vi "Teleop.vi"(10 "Match Info":T1={"Autonomous Elapsed Seconds"=0.0, "TeleOp Elapsed Seconds"=0.0, "Disabled Elapsed Seconds"=0.0, "Visited Autonomous"=FALSE, "Visited TeleOp"=FALSE, "Visited Disabled"=FALSE, "Autonomous Settings"={"Autonomous Style"=enum."Independent", "VI Refnum"=refnum}}, 11 "Call Context":T2) -> ()   [LabVIEW 2012]
doc: "This VI is called for each TeleOp packet received from the DS where the robot is not disabled. It is often used to read from the joysticks and update I/O or to update setpoints for timed control loops. It should complete and return within 20 milliseconds or it may miss DS packets."
uses:
  <vilib>/Rock Robotics/WPI/DriverStation/WPI_DriverStationDerivedRobotMode.ctl
  <vilib>/Rock Robotics/WPI/DriverStation/WPI_DriverStationMatch Info.ctl
  Robot Global Data.vi
  <vilib>/Rock Robotics/WPI/RobotDrive/WPI_RobotDriveGetSetRefNum.vi
panel:
  in  "Feeder Angle On Cannon In Minimum Position":dbl
  in  "Feeder Sit On Cannon?":bool=TRUE
  out "Cannon Angle (Relative to the Horizon)":dbl
  in  "reset":bool
  in  "Telescopic Toghether?":bool
  in  "Cannons Toghether?":bool
  in  "Cananot Toghether?":bool
  in  "2  Cananot (Climb)":dbl(slide) scale=-1.0..1.0
  in  "2  Telescopic(Climb)":dbl(slide) scale=-1.0..1.0
  in  "2 Cannons":dbl(slide) scale=-1.0..1.0
  in  "Flipper Servos":i32(knob) scale=0.0..170.0
  in  "Feeder Servos":i32(knob) scale=0.0..160.0
  in  "Climb Telescopic Right":dbl(slide) scale=-1.0..1.0
  in  "Climb Telescopic Left":dbl(slide) scale=-1.0..1.0
  in  "Transfer":dbl(slide) scale=-1.0..1.0
  in  "Canenet Left":dbl(slide) scale=-1.0..1.0
  in  "Canenet Right":dbl(slide) scale=-1.0..1.0
  in  "Conveyer Belt":dbl(slide) scale=-1.0..1.0
  in  "zAvit":dbl(slide) scale=-1.0..1.0
  in  "First Cannon":dbl(slide) scale=-1.0..1.0
  in  "Second Cannon":dbl(slide) scale=-1.0..1.0
  in  "Y axis value":dbl(slide) scale=-1.0..1.0
  in  "X axis value":dbl(slide) scale=-1.0..1.0
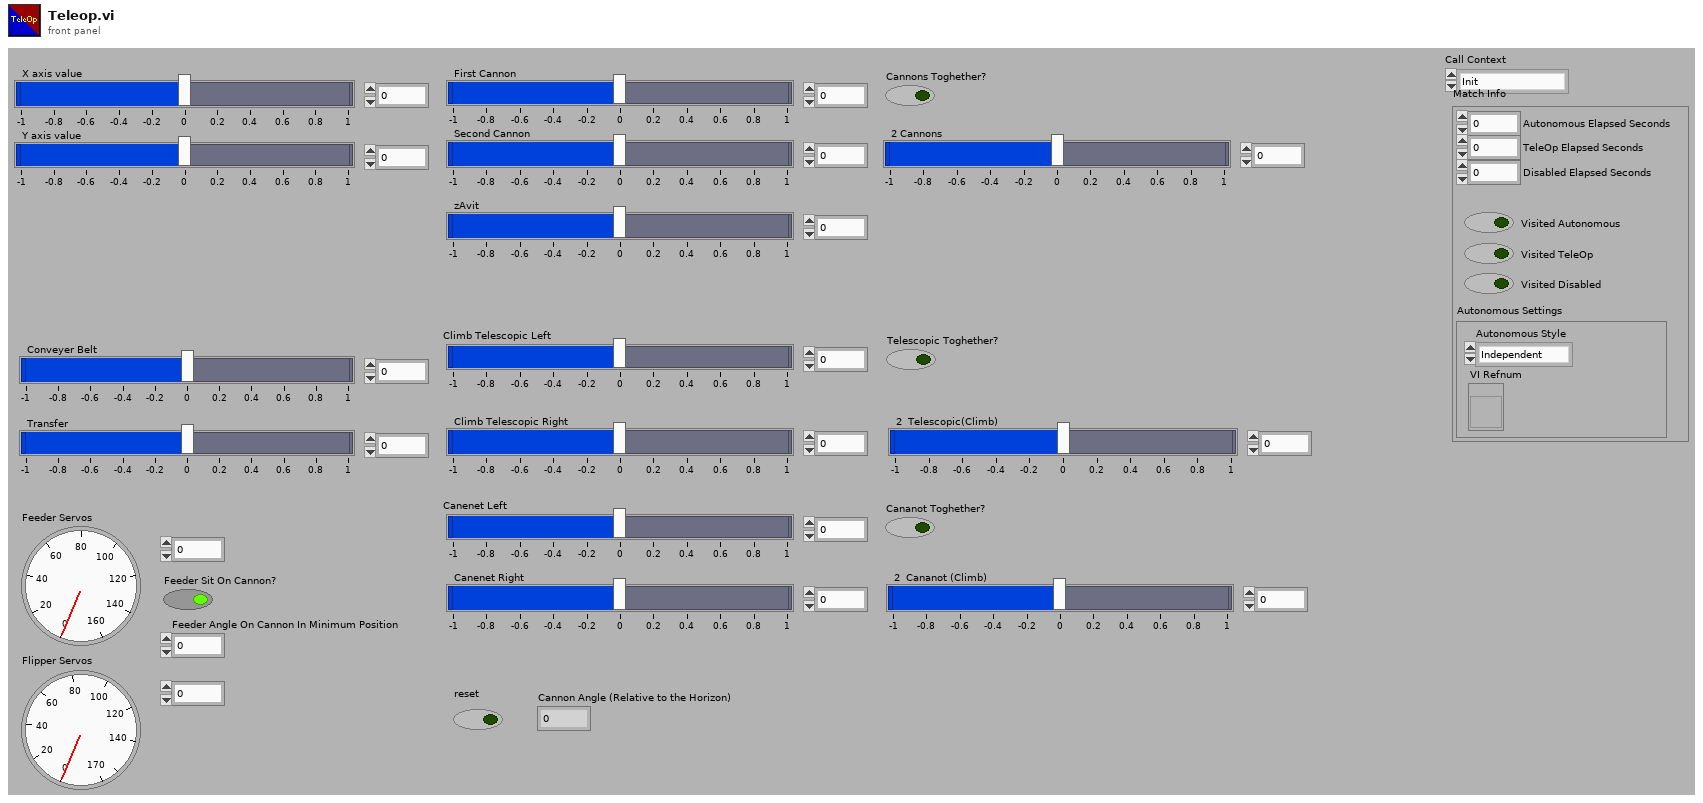
[diagram p1: front panel]
types:
  T1 = typedef "WPI_DriverStationMatch Info.ctl" = cluster{"Autonomous Elapsed Seconds":dbl, "TeleOp Elapsed Seconds":dbl, "Disabled Elapsed Seconds":dbl, "Visited Autonomous":bool, "Visited TeleOp":bool, "Visited Disabled":bool, "Autonomous Settings":cluster{"Autonomous Style":enum16{"Iterative", "Independent"}, "VI Refnum":refnum<vi>}}
  T2 = typedef "WPI_DriverStationDerivedRobotMode.ctl" = enum16{"Init", "Execute", "Stop"}
  T3 = typedef "WPI_AnalogChannelDevRef.ctl" = cluster{"DevStatus":errorcluster, "Analog Module":T4, "Analog Channel":T5}
  T4 = typedef "FPGA_TypedefAnalogModule.ctl" = enum16{"Analog Module 1", "Analog Module 2"}
  T5 = typedef "FPGA_AIChannel.ctl" = enum8{"AI 1", "AI 2", "AI 3", "AI 4", "AI 5", "AI 6", "AI 7", "AI 8", "Invalid"}
  T6 = typedef "WPI_DigitalInputDevRef.ctl" = cluster{"DevStatus":errorcluster, "DIO Channel":T7, "Digital Module":T8}
  T7 = typedef "FPGA_DIOChannel.ctl" = enum8{"DIO 1", "DIO 2", "DIO 3", "DIO 4", "DIO 5", "DIO 6", "DIO 7", "DIO 8", "DIO 9", "DIO 10", "DIO 11", "DIO 12", "DIO 13", "DIO 14", "Invalid"}
  T8 = typedef "FPGA_TypedefDigitalModule.ctl" = enum16{"Digital Module 1", "Digital Module 2"}
  T9 = typedef "WPI_MotorControlDeviceRef.ctl" = cluster{"DeviceStatus":errorcluster, "Type":enum16{"PWM", "CAN"}, "PWM":cluster{"Digital Module":T8, "PWM Channel":T10, "DeadBand":T11}, "CAN":cluster{"Device Number":u8, "Control Mode":T12, "Semaphore":T13, "Max Vout":dbl}, "Invert":bool, "TransformRef":T14, "InvTransformRef":T14}
  T10 = typedef "FPGA_DIOPWMChannel.ctl" = enum8{"PWM 1", "PWM 2", "PWM 3", "PWM 4", "PWM 5", "PWM 6", "PWM 7", "PWM 8", "PWM 9", "PWM 10", "Invalid"}
  T11 = typedef "WPI_PWMDeadband.ctl" = cluster{"Name":string, "maxPositivePwm":i32, "minPositivePwm":i32, "centerPwm":i32, "maxNegativePwm":i32, "minNegativePwm":i32, "angularRange":u16}
  T12 = typedef "WPI_CANJaguar_ControlMode.ctl" = enum8{"Percent VBus", "Current", "Speed", "Position", "Voltage"}
  T13 = typedef "Semaphore RefNum" = refnum<k1>
  T14 = typedef "WPI_PWMTransform_ConPane.ctl" = refnum<vi>
  T15 = typedef "WPI_ServoDeviceRef.ctl" = cluster{"DeviceStatus":errorcluster, "Digital Module":T8, "PWM Channel":T10, "DeadBand":T11}
  T16 = typedef "WPI_RobotDriveDevRef.ctl" = cluster{"DevStatus":errorcluster, "Motors[]":T9[], "Square Inputs":bool, "Max Output":dbl, "Isochronous":bool}
  T17 = typedef "WPI_RelayDevRef.ctl" = cluster{"DevStatus":errorcluster, "Relay Channel":T18, "Digital Module":T8, "Relay Direction":T19}
  T18 = typedef "FPGA_DIORelayChannel.ctl" = enum8{"Relay 1", "Relay 2", "Relay 3", "Relay 4", "Relay 5", "Relay 6", "Relay 7", "Relay 8", "Invalid"}
  T19 = typedef "WPI_RelayDirection.ctl" = enum16{"Both directions", "Forward only", "Reverse only"}
  T20 = typedef "WPI_RelayValue.ctl" = enum16{"Off", "On", "Forward", "Reverse"}
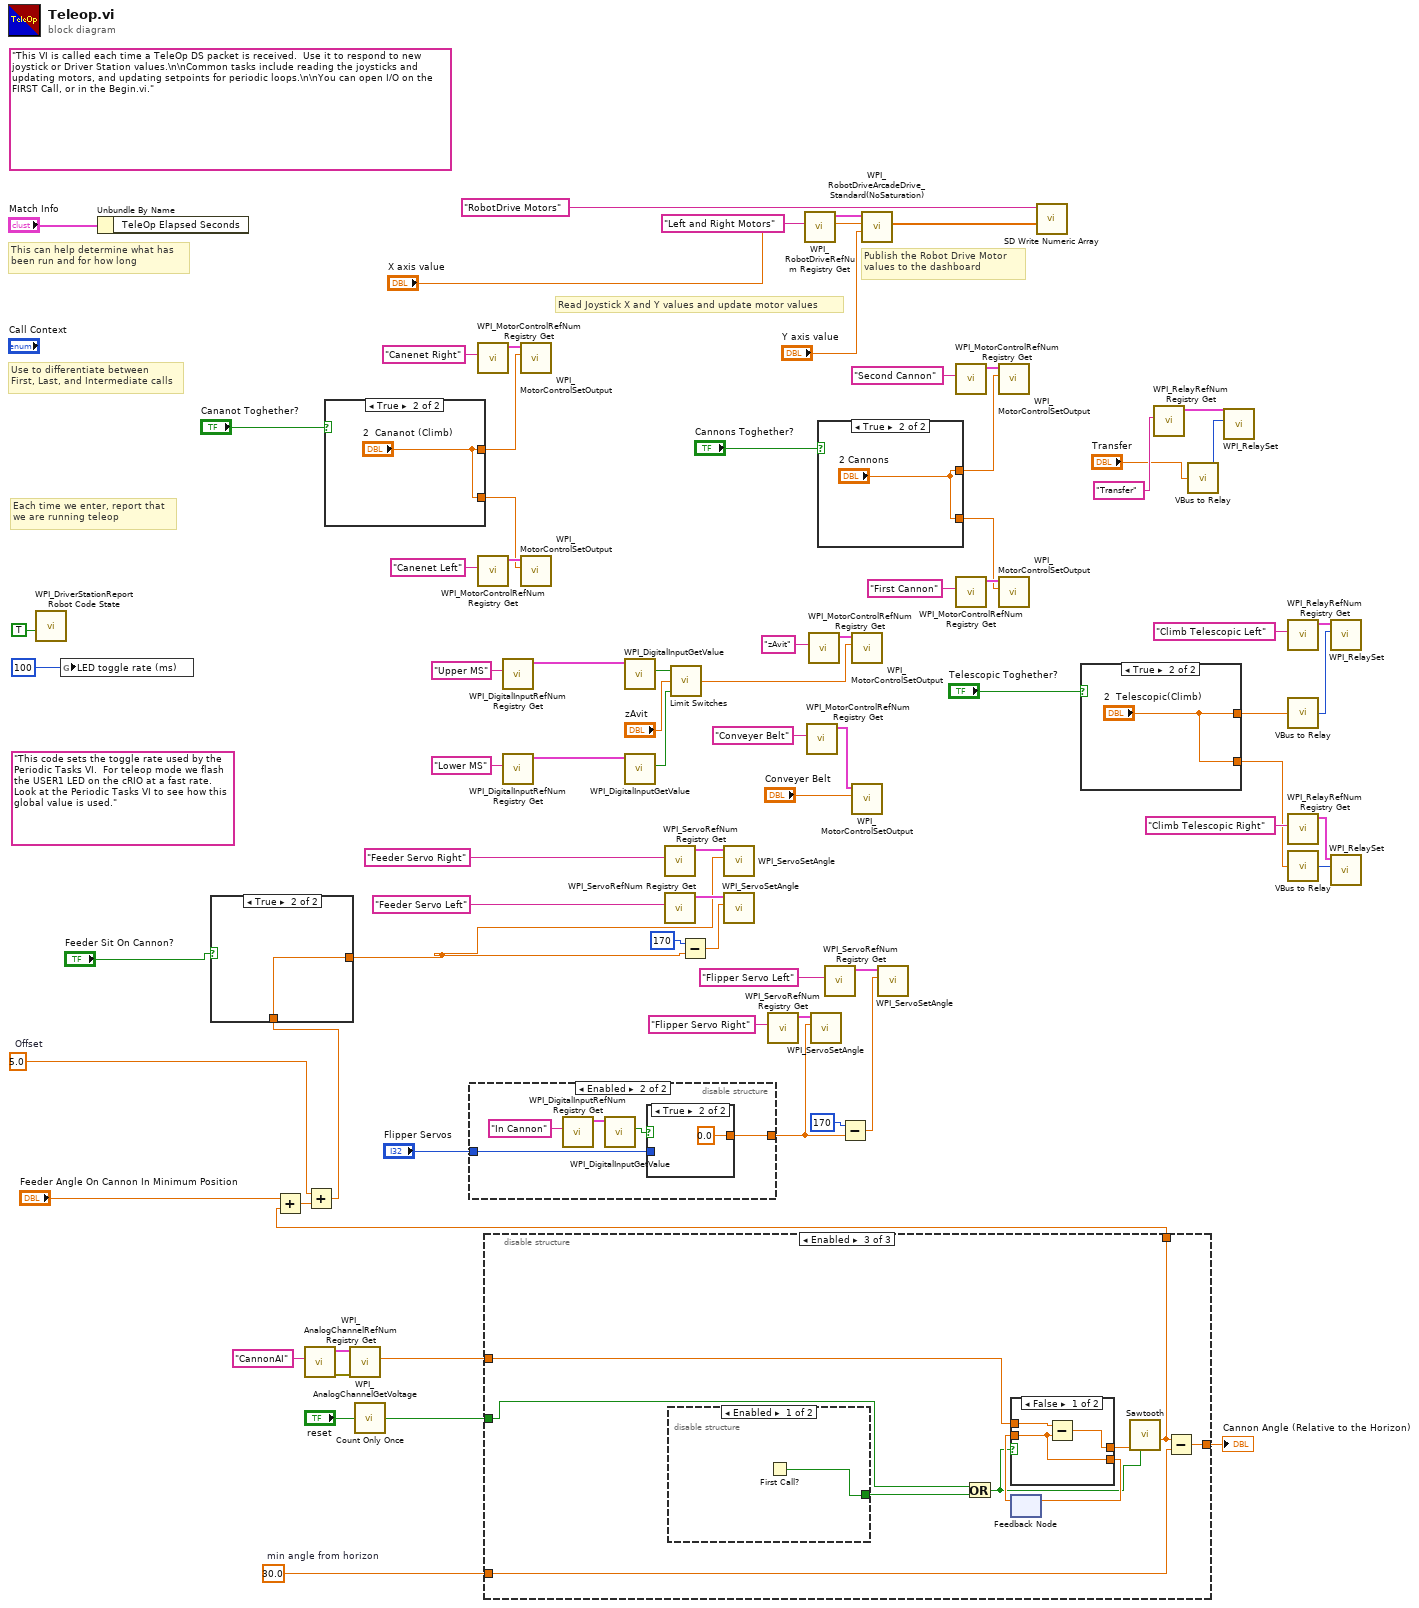
[diagram p0: block diagram]
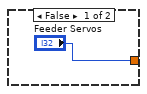
[diagram p4: hidden frame]
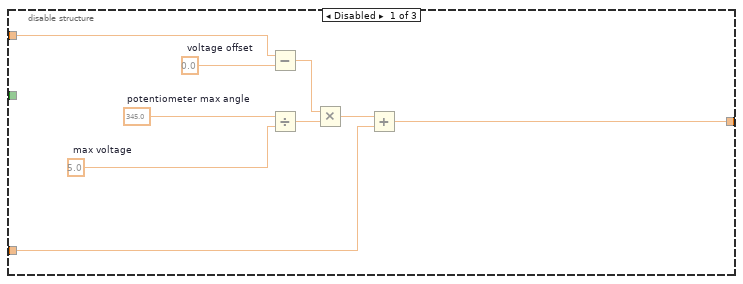
[diagram p5: hidden frame]
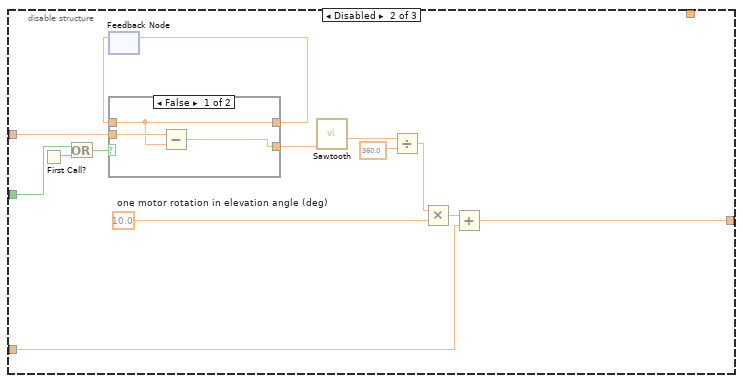
[diagram p6: hidden frame]
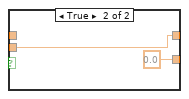
[diagram p7: hidden frame]
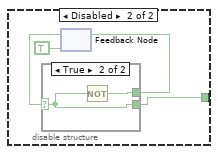
[diagram p8: hidden frame]
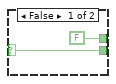
[diagram p9: hidden frame]
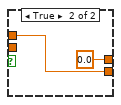
[diagram p10: hidden frame]
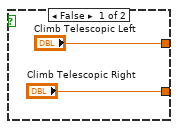
[diagram p11: hidden frame]
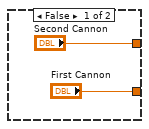
[diagram p12: hidden frame]
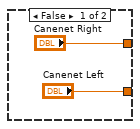
[diagram p13: hidden frame]
diagram:
  w4 = 5.0  # Offset
  w19 = 30.0  # min angle from horizon
  (unwired) "This code sets the toggle rate used by the Periodic Tasks VI.  For teleop mode we flash the USER1 LED on the cRIO at a fast rate.  Look at the Periodic Tasks VI to see how this global value is used."
  (unwired) "This VI is called each time a TeleOp DS packet is received.  Use it to respond to new joystick or Driver Station values.\n\nCommon tasks include reading the joysticks and updating motors, and updating setpoints for periodic loops.\n\nYou can open I/O on the FIRST Call, or in the Begin.vi."
  # "Publish the Robot Drive Motor\nvalues to the dashboard"
  # "Each time we enter, report that\nwe are running teleop"
  # "Use to differentiate between\nFirst, Last, and Intermediate calls"
  # "This can help determine what has\nbeen run and for how long"
  # "Read Joystick X and Y values and update motor values"
  n1 = call <vilib>:"WPI_DriverStationReport Robot Code State.vi"("TeleOp"=TRUE ("Autonomous")) -> ()  [unwired: 10 in, 1 out]
  n2 = global write "Robot Global Data.vi" "LED toggle rate (ms)"(u32 100 ("LED ms toggle rate")) -> ()
  n3 = Unbundle By Name("Match Info") -> ()  [unwired: 1 out]
  n4 = call <vilib>:"WPI_AnalogChannelRefNum Registry Get.vi"("refnum name"="CannonAI") -> ("error out"=w20:errorcluster, "AIDeviceRef"=w22:T3)  [unwired: 9 in]
  n5 = case shown="True" "Cananot Toghether?" {
    tunnel: ["Canenet Right" "2  Cananot (Climb)"] -> w33
    tunnel: ["Canenet Left" "2  Cananot (Climb)"] -> w32
    frame False {
    }
    frame True {
    }
  }
  n6 = call <vilib>:"WPI_AnalogChannelGetVoltage.vi"("error in (no error)"=w20, "AIDeviceRef"=w22) -> ("Voltage"=w21:dbl)  [unwired: 7 in, 2 out]
  n7 = call "Count Only Once.vi"("InValue"="reset") -> ("Result"=w17:bool)
  n8 = disable-structure shown="Enabled" {
    disable-tunnel: [w82 w87] -> w2
    disable-tunnel: "Flipper Servos" -> [w82 w83]
    frame Disabled {
    }
    frame Enabled {
      n9 = call <vilib>:"WPI_DigitalInputRefNum Registry Get.vi"("refnum name"="In Cannon") -> ("DigitalInputDevRef"=w86:T6)  [unwired: 9 in, 1 out]
      n10 = call <vilib>:"WPI_DigitalInputGetValue.vi"("DigitalInputDevRef"=w86) -> ("Value"=w84:bool)  [unwired: 8 in, 2 out]
      n11 = case shown="True" w84 {
        tunnel: [w88 0.0] -> w87
        tunnel: w83 -> [w88 _]
        frame False {
        }
        frame True {
        }
      }
    }
  }
  n12 = call <vilib>:"WPI_MotorControlRefNum Registry Get.vi"("refnum name"="Canenet Right") -> ("MotorControlDevRef"=w51:T9)  [unwired: 9 in, 1 out]
  n13 = call <vilib>:"WPI_MotorControlRefNum Registry Get.vi"("refnum name"="Canenet Left") -> ("MotorControlDevRef"=w50:T9)  [unwired: 9 in, 1 out]
  n14 = disable-structure shown="Enabled" {
    disable-tunnel: w21 -> [w98 w105 w125]
    disable-tunnel: [w93 w111 w126] -> w10
    disable-tunnel: w19 -> [w90 w112 w127]
    disable-tunnel: w17 -> [_ w100 w120]
    disable-tunnel: [_ _ w118] -> w7
    frame Disabled {
      w91 = 0.0  # voltage offset
      w95 = 5.0  # max voltage
      w96 = 345.0  # potentiometer max angle
      n15 = Subtract(x=w98, y=w91) -> (x-y=w92:dbl)
      n16 = Divide(x=w96, y=w95) -> (x/y=w94:dbl)
      n17 = Multiply(x=w92, y=w94) -> (x*y=w97:dbl)
      n18 = Add(x=w97, y=w90) -> (x+y=w93:dbl)
    }
    frame Disabled {
      w106 = 10.0  # one motor rotation in elevation angle (deg)
      n19 = First Call?() -> (First Call?: T/F=w101:bool)
      n20 = Or(x=w100, y=w101) -> (x .or. y?=w99:bool)
      n21 = feedback #1() -> (w103:dbl)  [unwired: 1 in]
      n22 = case shown="False" w99 {
        tunnel: w105 -> [w115 w117]
        tunnel: [w114 w117] -> w104
        tunnel: w103 -> [w114 _]
        tunnel: [w113 0.0] -> w102
        frame False {
          n23 = Subtract(x=w115, y=w114) -> (x-y=w113:dbl)
        }
        frame True {
        }
      }
      n24 = feedback-in #1(w104) -> ()
      n25 = call "Sawtooth.vi"("Voltage"=w102) -> ("Absolute Angle (deg)"=w110:dbl)  [unwired: 8 in, 2 out]
      n26 = Divide(x=w110, y=360.0) -> (x/y=w108:dbl)
      n27 = Multiply(x=w108, y=w106) -> (x*y=w107:dbl)
      n28 = Add(x=w107, y=w112) -> (x+y=w111:dbl)
    }
    frame Enabled {
      n29 = disable-structure shown="Enabled" {
        disable-tunnel: [w128 w130] -> w121
        frame Enabled {
          n30 = First Call?() -> (First Call?: T/F=w128:bool)
        }
        frame Disabled {
          n31 = feedback #2(TRUE) -> (w132:bool)
          n32 = case shown="True" w132 {
            selector: w132 -> [w134 w136]
            tunnel: [w134 w136] -> w130
            tunnel: [FALSE w135] -> w129
            frame False {
            }
            frame True {
              n33 = Not(x=w136) -> (.not. x?=w135:bool)
            }
          }
          n34 = feedback-in #2(w129) -> ()
        }
      }
      n35 = Or(x=w120, y=w121) -> (x .or. y?=w119:bool)
      n36 = feedback #3() -> (w123:dbl)  [unwired: 1 in]
      n37 = case shown="False" w119 {
        tunnel: w125 -> [w139 w141]
        tunnel: [w138 w141] -> w124
        tunnel: w123 -> [w138 _]
        tunnel: [w137 0.0] -> w122
        frame False {
          n38 = Subtract(x=w139, y=w138) -> (x-y=w137:dbl)
        }
        frame True {
        }
      }
      n39 = feedback-in #3(w124) -> ()
      n40 = call "Sawtooth.vi"("Reintalize?"=w119, "Voltage"=w122) -> ("Absolute Angle (deg)"=w118:dbl)  [unwired: 7 in, 2 out]
      n41 = Subtract(x=w118, y=w127) -> (x-y=w126:dbl)
    }
  }
  "Cannon Angle (Relative to the Horizon)" <- w10
  n42 = Add(x="Feeder Angle On Cannon In Minimum Position", y=w7) -> (x+y=w5:dbl)
  n43 = Add(x=w4, y=w5) -> (x+y=w3:dbl)
  n44 = case shown="True" "Feeder Sit On Cannon?" {
    tunnel: ["Feeder Servos" w143] -> w8
    tunnel: w3 -> [_ w143]
    frame False {
    }
    frame True {
    }
  }
  n45 = call <vilib>:"WPI_DigitalInputRefNum Registry Get.vi"("refnum name"="Upper MS") -> ("DigitalInputDevRef"=w16:T6)  [unwired: 9 in, 1 out]
  n46 = call <vilib>:"WPI_DigitalInputRefNum Registry Get.vi"("refnum name"="Lower MS") -> ("DigitalInputDevRef"=w13:T6)  [unwired: 9 in, 1 out]
  n47 = call <vilib>:"WPI_MotorControlSetOutput.vi"("Output"=w33, "MotorControlDevRef"=w51) -> ()  [unwired: 7 in, 3 out]
  n48 = call <vilib>:"WPI_MotorControlSetOutput.vi"("Output"=w32, "MotorControlDevRef"=w50) -> ()  [unwired: 7 in, 3 out]
  n49 = call <vilib>:"WPI_DigitalInputGetValue.vi"("DigitalInputDevRef"=w16) -> ("Value"=w11:bool)  [unwired: 8 in, 2 out]
  n50 = call <vilib>:"WPI_DigitalInputGetValue.vi"("DigitalInputDevRef"=w13) -> ("Value"=w12:bool)  [unwired: 8 in, 2 out]
  n51 = call <vilib>:"WPI_ServoRefNum Registry Get.vi"("refnum name"="Feeder Servo Right") -> ("ServoDeviceRef"=w68:T15)  [unwired: 9 in, 1 out]
  n52 = call <vilib>:"WPI_ServoRefNum Registry Get.vi"("refnum name"="Feeder Servo Left") -> ("ServoDeviceRef"=w69:T15)  [unwired: 9 in, 1 out]
  n53 = call "Limit Switches.vi"("Backward Limit Switch"=w12, "VBus in"="zAvit", "Forward Limit Switch"=w11) -> ("VBus out"=w24:dbl)
  n54 = Subtract(x=170, y=w8) -> (x-y=w35:dbl)
  n55 = call <vilib>:"WPI_ServoSetAngle.vi"("Angle"=w8, "ServoDeviceRef"=w68) -> ()  [unwired: 8 in, 2 out]
  n56 = call <vilib>:"WPI_ServoSetAngle.vi"("Angle"=w35, "ServoDeviceRef"=w69) -> ()  [unwired: 8 in, 2 out]
  n57 = call <vilib>:"WPI_ServoRefNum Registry Get.vi"("refnum name"="Flipper Servo Right") -> ("ServoDeviceRef"=w66:T15)  [unwired: 9 in, 1 out]
  n58 = call <vilib>:"WPI_RobotDriveRefNum Registry Get.vi"("refnum name"="Left and Right Motors") -> ("RobotDriveDevRef"=w76:T16)  [unwired: 1 in, 9 out]
  n59 = call <vilib>:"WPI_MotorControlRefNum Registry Get.vi"("refnum name"="Conveyer Belt") -> ("MotorControlDevRef"=w54:T9)  [unwired: 9 in, 1 out]
  n60 = call <vilib>:"WPI_MotorControlRefNum Registry Get.vi"("refnum name"="zAvit") -> ("MotorControlDevRef"=w57:T9)  [unwired: 9 in, 1 out]
  n61 = call <vilib>:"WPI_ServoSetAngle.vi"("Angle"=w2, "ServoDeviceRef"=w66) -> ()  [unwired: 8 in, 2 out]
  n62 = case shown="True" "Cannons Toghether?" {
    tunnel: ["First Cannon" "2 Cannons"] -> w30
    tunnel: ["Second Cannon" "2 Cannons"] -> w29
    frame False {
    }
    frame True {
    }
  }
  n63 = call <vilib>:"WPI_ServoRefNum Registry Get.vi"("refnum name"="Flipper Servo Left") -> ("ServoDeviceRef"=w67:T15)  [unwired: 9 in, 1 out]
  n64 = Subtract(x=170, y=w2) -> (x-y=w34:dbl)
  n65 = call <vilib>:"WPI_MotorControlSetOutput.vi"("Output"=w24, "MotorControlDevRef"=w57) -> ()  [unwired: 7 in, 3 out]
  n66 = call <vilib>:"WPI_MotorControlSetOutput.vi"("Output"="Conveyer Belt", "MotorControlDevRef"=w54) -> ()  [unwired: 7 in, 3 out]
  n67 = call <vilib>:"WPI_RobotDriveArcadeDrive_Standard(NoSaturation).vi"("Y axis value"="Y axis value", "X axis value"="X axis value", "RobotDriveDevRef"=w76) -> ("Motor Values"=w72:dbl[])  [unwired: 1 in, 7 out]
  n68 = call <vilib>:"WPI_ServoSetAngle.vi"("Angle"=w34, "ServoDeviceRef"=w67) -> ()  [unwired: 8 in, 2 out]
  n69 = call <vilib>:"WPI_MotorControlRefNum Registry Get.vi"("refnum name"="Second Cannon") -> ("MotorControlDevRef"=w58:T9)  [unwired: 9 in, 1 out]
  n70 = call <vilib>:"WPI_MotorControlRefNum Registry Get.vi"("refnum name"="First Cannon") -> ("MotorControlDevRef"=w61:T9)  [unwired: 9 in, 1 out]
  n71 = call <vilib>:"WPI_MotorControlSetOutput.vi"("Output"=w29, "MotorControlDevRef"=w58) -> ()  [unwired: 7 in, 3 out]
  n72 = call <vilib>:"WPI_MotorControlSetOutput.vi"("Output"=w30, "MotorControlDevRef"=w61) -> ()  [unwired: 7 in, 3 out]
  n73 = call <vilib>:"SD Write Numeric Array.vi"("Numeric Array"=w72, "Name"="RobotDrive Motors") -> ()  [unwired: 8 in, 2 out]
  n74 = case shown="True" "Telescopic Toghether?" {
    tunnel: ["Climb Telescopic Left" "2  Telescopic(Climb)"] -> w27
    tunnel: ["Climb Telescopic Right" "2  Telescopic(Climb)"] -> w26
    frame False {
    }
    frame True {
    }
  }
  n75 = call <vilib>:"WPI_RelayRefNum Registry Get.vi"("refnum name"="Transfer") -> ("RelayDevRef"=w48:T17)  [unwired: 9 in, 1 out]
  n76 = call "VBus to Relay.vi"("Motor VBus"="Transfer") -> ("RelayValue"=w45:T20)  [unwired: 3 in]
  n77 = call <vilib>:"WPI_RelaySet.vi"("RelayValue"=w45, "RelayDevRef"=w48) -> ()  [unwired: 8 in, 2 out]
  n78 = call <vilib>:"WPI_RelayRefNum Registry Get.vi"("refnum name"="Climb Telescopic Left") -> ("RelayDevRef"=w43:T17)  [unwired: 9 in, 1 out]
  n79 = call "VBus to Relay.vi"("Motor VBus"=w27) -> ("RelayValue"=w44:T20)  [unwired: 3 in]
  n80 = call <vilib>:"WPI_RelayRefNum Registry Get.vi"("refnum name"="Climb Telescopic Right") -> ("RelayDevRef"=w42:T17)  [unwired: 9 in, 1 out]
  n81 = call "VBus to Relay.vi"("Motor VBus"=w26) -> ("RelayValue"=w41:T20)  [unwired: 3 in]
  n82 = call <vilib>:"WPI_RelaySet.vi"("RelayValue"=w44, "RelayDevRef"=w43) -> ()  [unwired: 8 in, 2 out]
  n83 = call <vilib>:"WPI_RelaySet.vi"("RelayValue"=w41, "RelayDevRef"=w42) -> ()  [unwired: 8 in, 2 out]
